vi "Spawn Primary Weapon.vi"(11 "Arilou in":refnum<class "Arilou.lvclass">) -> (2 "New Elements":refnum<class "Element.lvclass">[](array[class]), 3 "Arilou out":refnum<class "Arilou.lvclass">)   [LabVIEW 2021, in "Arilou.lvclass"]
uses:
  Arilou.lvclass
  C:/dev/LabVIEW/LabMelee/Source/Application Specific/Element/Element.lvclass
  Element/Element.lvclass
  Element/Element.lvclass/Element.ctl
  Motion/Motion.lvclass/Motion.ctl
  Vector 2D/Vector 2D.lvclass/Vector 2D.ctl
  Weapons/Laser/Laser.lvclass
  Vector 2D/Vector 2D.lvclass
  Ship/Ship.lvclass
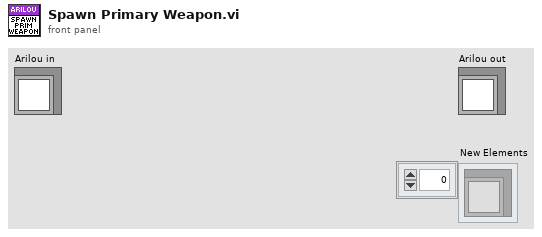
[diagram p1: front panel]
types:
  T1 = typedef "Main Controller Actor.lvclass/Player.ctl" = enum16{"1", "2"}
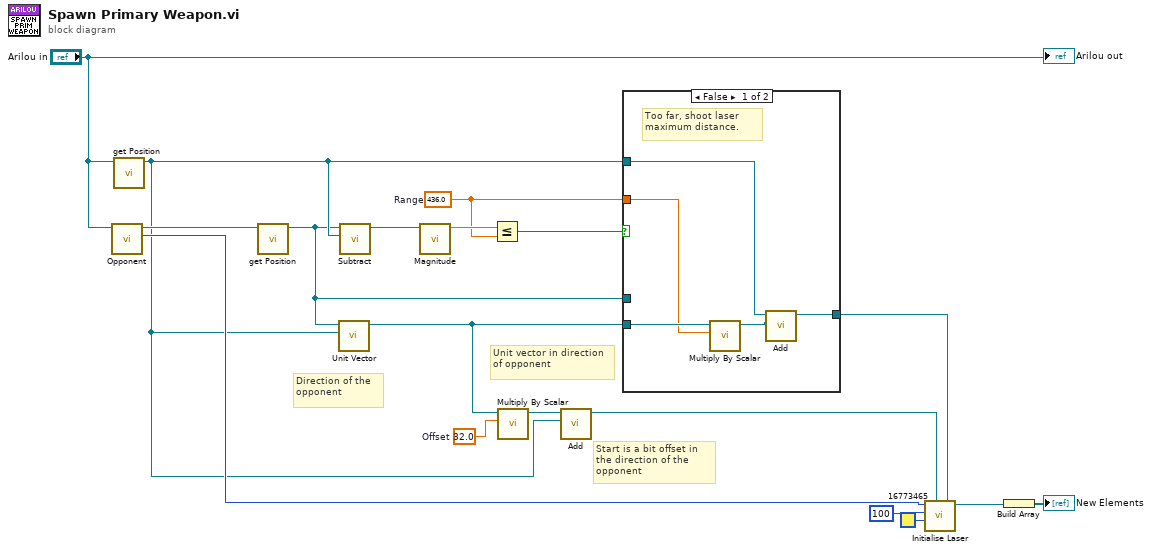
[diagram p0: block diagram]
diagram:
  w1 = sgl 436.0  # Range
  w3 = sgl 32.0  # Offset
  # "Unit vector in direction of opponent"
  # "Start is a bit offset in the direction of the opponent"
  # "Direction of the opponent"
  n1 = call "Opponent.vi"("Element in"="Arilou in") -> ("This Player"=w13:T1, "Opponent out"=w14:refnum<class "Element.lvclass">)  [unwired: 9 in]
  n2 = call "get Position.vi"("Element in"="Arilou in") -> ("Position"=w6:refnum<class "Vector 2D.lvclass">)  [unwired: 10 in]
  n3 = call "get Position.vi"("Element in"=w14) -> ("Position"=w5:refnum<class "Vector 2D.lvclass">)  [unwired: 10 in]
  n4 = call "Unit Vector.vi"("Position 2"=w6, "Position 1"=w5) -> ("Unit Vector In Direction"=w9:refnum<class "Vector 2D.lvclass">)  [unwired: 9 in]
  n5 = call "Subtract.vi"("B"=w6, "A"=w5) -> ("A-B"=w7:refnum<class "Vector 2D.lvclass">)  [unwired: 9 in]
  n6 = call "Magnitude.vi"("A"=w7) -> ("Magnitude"=w12:sgl)  [unwired: 10 in]
  n7 = Less Or Equal?(x=w12, y=w1) -> (x <= y?=w11:bool)
  n8 = call "Multiply By Scalar.vi"("x"=w3, "A"=w9) -> ("Ax"=w4:refnum<class "Vector 2D.lvclass">)  [unwired: 9 in]
  n9 = call "Add.vi"("B"=w6, "A"=w4) -> ("A+B"=w2:refnum<class "Vector 2D.lvclass">)  [unwired: 9 in]
  n10 = case shown="False" w11 {
    tunnel: w5 -> [_ w24]
    tunnel: w6 -> [w21 _]
    tunnel: w9 -> [w22 _]
    tunnel: [w23 w24] -> w8
    tunnel: w1 -> [w19 _]
    frame False {
      # "Too far, shoot laser maximum distance."
      n11 = call "Multiply By Scalar.vi"("x"=w19, "A"=w22) -> ("Ax"=w20:refnum<class "Vector 2D.lvclass">)  [unwired: 9 in]
      n12 = call "Add.vi"("B"=w20, "A"=w21) -> ("A+B"=w23:refnum<class "Vector 2D.lvclass">)  [unwired: 9 in]
    }
    frame True {
      # "Ships is in distance. Start a bit offset , just end directly at the target"
    }
  }
  n13 = call "Initialise Laser.vi"("Endpoint"=w8, "Origin"=w2, "Colour"=u32 16773465, "Damage"=100, "Player"=w13) -> ("Laser out"=w17:refnum<class "Laser.lvclass">)  [unwired: 6 in]
  n14 = Build Array(w17) -> (→"New Elements":refnum<class "Laser.lvclass">[])
  "Arilou out" <- "Arilou in"
